vi "enableOrDisable.vi"(8 "error in (no error)":errorcluster, 10 "Enable?":bool, 11 "Control References":refnum<vi>[](array[refnum])) -> (0 "error out":errorcluster)   [LabVIEW 2019]
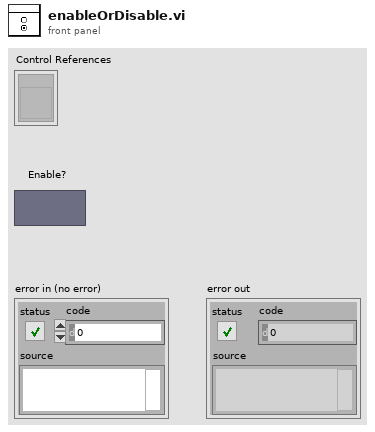
[diagram p1: front panel]
types:
  T1 = enum8{"Enabled", "Disabled", "Disabled and Grayed Out"}
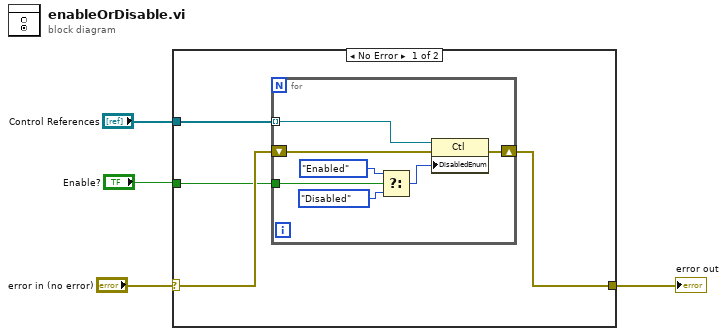
[diagram p0: block diagram]
diagram:
  n1 = case shown="No Error" "error in (no error)" {
    selector: "error in (no error)" -> [w8 w16]
    tunnel: [w7 w16] -> w4
    tunnel: "Control References" -> [w6 _]
    tunnel: "Enable?" -> [w5 _]
    frame No Error {
      n2 = for {
        shift-right: [w14] -> w7
        shift-left: w8 -> [w15]
        tunnel: w6 -> [w13] mode=indexing
        tunnel: w5 -> [w9]
        n3 = Select(t=T1."Enabled" ("Disabled"), s=w9, f=T1."Disabled" ("Disabled")) -> (s? t:f=w10:T1)
        n4 = property class="Ctl"(reference=w13, error in=w15, "DisabledEnum"=w10) -> (error out=w14:errorcluster)  [unwired: 1 out]
      }
    }
    frame Error {
    }
  }
  "error out" <- w4
